vi "Test_Convert_Distance_to_Flywheel_Velocity.vi"() -> ()   [LabVIEW 2019]
panel:
  out "distance":dbl
  out "velocity":dbl
  in  "angle":dbl=30.0
  in  "terminal height":dbl=90.5
  out "Numeric":i32
  out "velocities":dbl[](array[numeric])
  out "distances":dbl[](array[numeric])
  out "Test Plot":cluster{dbl[], dbl[]}(graph)
  in  "StopValue":dbl=300.0
  in  "StartValue":dbl
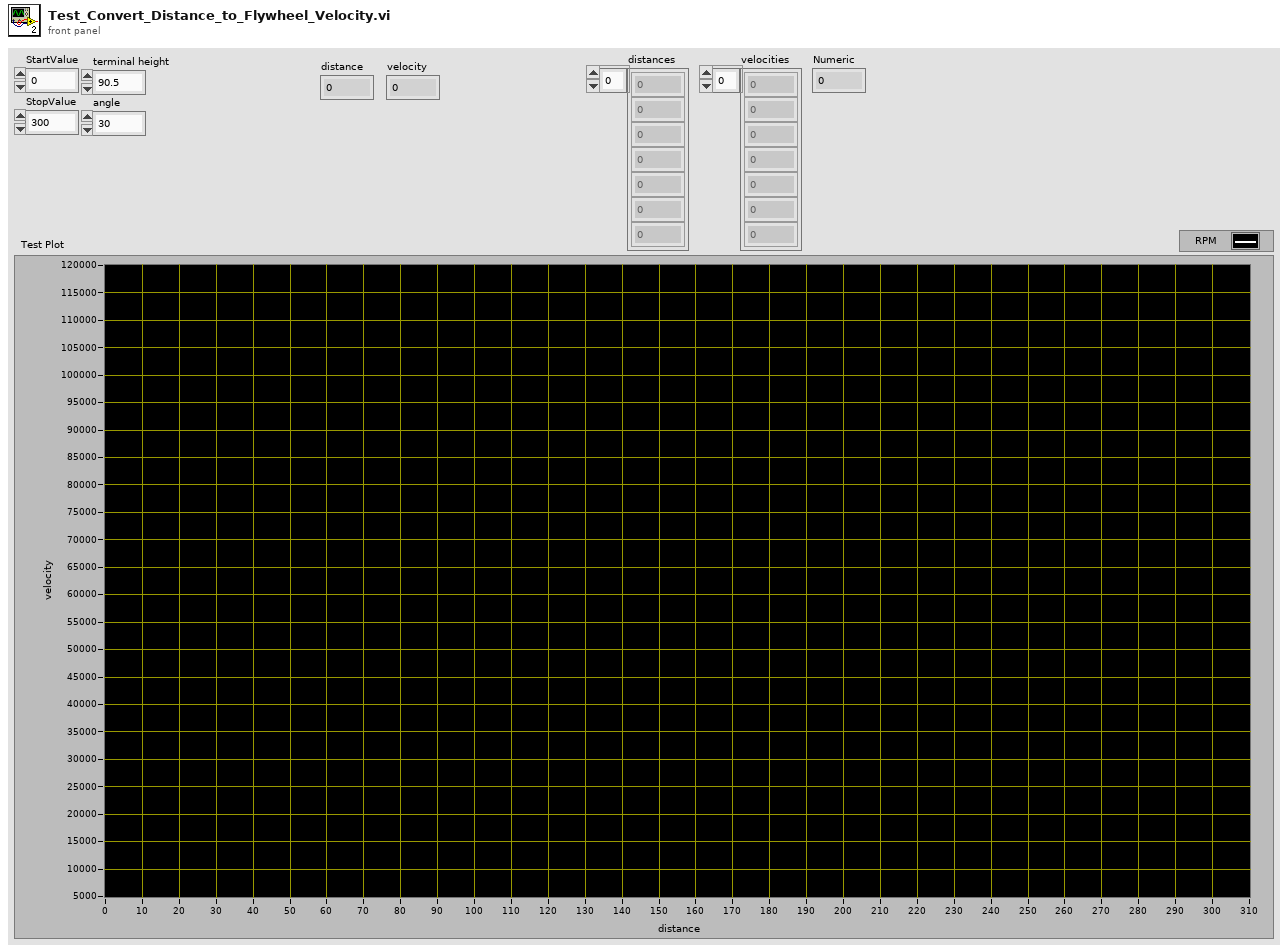
[diagram p1: front panel]
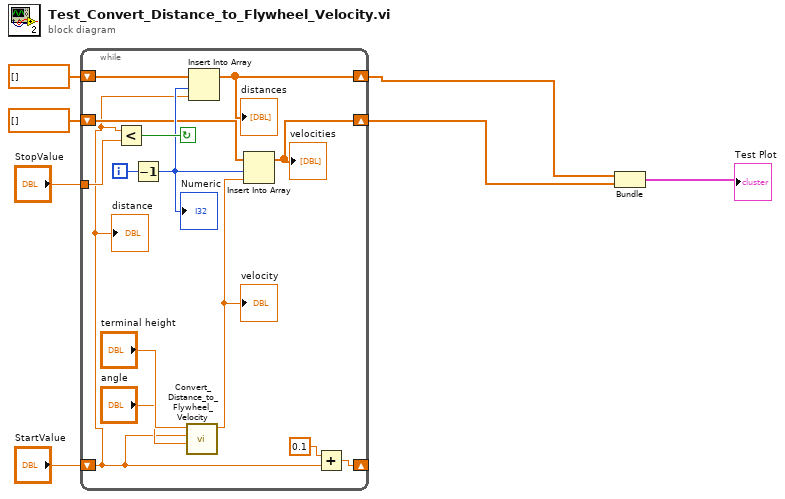
[diagram p0: block diagram]
diagram:
  n1 = while {
    shift-right: [w20] -> _
    shift-left: "StartValue" -> [w8]
    tunnel: "StopValue" -> [w19]
    shift-right: [w13] -> w3
    shift-left: dbl[] [] -> [w15]
    shift-right: [w12] -> w2
    shift-left: dbl[] [] -> [w14]
    i -> [w17]
    stop <- w18 continue-if-true
    n2 = Less?(x=w8, y=w19) -> (x < y?=w18:bool)
    n3 = Decrement(x=w17) -> (x-1=w16:i32)
    "Numeric" <- w16
    n4 = call "Convert_Distance_to_Flywheel_Velocity.vi"("angle"="angle", "distance"=w8, "terminal height"="terminal height") -> ("velocity"=w9:dbl)  [unwired: 8 in]
    "velocity" <- w9
    n5 = Insert Into Array(array=w15, index=w16, new element=w8) -> (w13:dbl[])
    "distances" <- w13
    n6 = Insert Into Array(array=w14, index=w16, new element=w9) -> (w12:dbl[])
    "velocities" <- w12
    n7 = Add(x=0.1, y=w8) -> (x+y=w20:dbl)
    "distance" <- w8
  }
  n8 = Bundle(w3, w2) -> (→"Test Plot":cluster{dbl[], dbl[]})  [unwired: 1 in]
